vi "collectResults.vi"(6 "Images to Collect":i32, 8 "error in (no error)":errorcluster, 9 "Enum":T1(ring), 10 "ImageData":T2, 11 "ImageAnalyser in":refnum<class "ImageAnalyser.lvclass">) -> (0 "error out":errorcluster, 2 "finished?":bool, 3 "ImageAnalyser out":refnum<class "ImageAnalyser.lvclass">)   [LabVIEW 2011, in "Tools.lvlib" / "Imaging.lvlib" / "ImageAnalyser.lvclass"]
uses:
  ImageAnalyser.lvclass
  ImageAnalyser.lvclass/ImageAnalyser.ctl
  AbsorptionAnalyser/AbsorptionAnalyser.lvclass
  FluorescenceAnalyser/FluorescenceAnalyser.lvclass
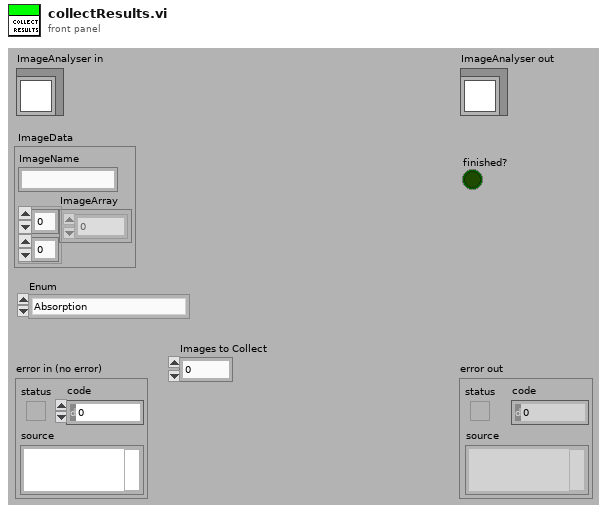
[diagram p1: front panel]
types:
  T1 = enum16{"Absorption", "Fluorescence", "Light Sheet", "Dark Ground"}
  T2 = cluster{"ImageName":string, "ImageArray":sgl[][]}
  T3 = cluster{"Name":string, "Results":dbl[], "AnalysisType":string}
  T4 = cluster{"Name":string, "Results":dbl[], "AnalysisType":string}[]
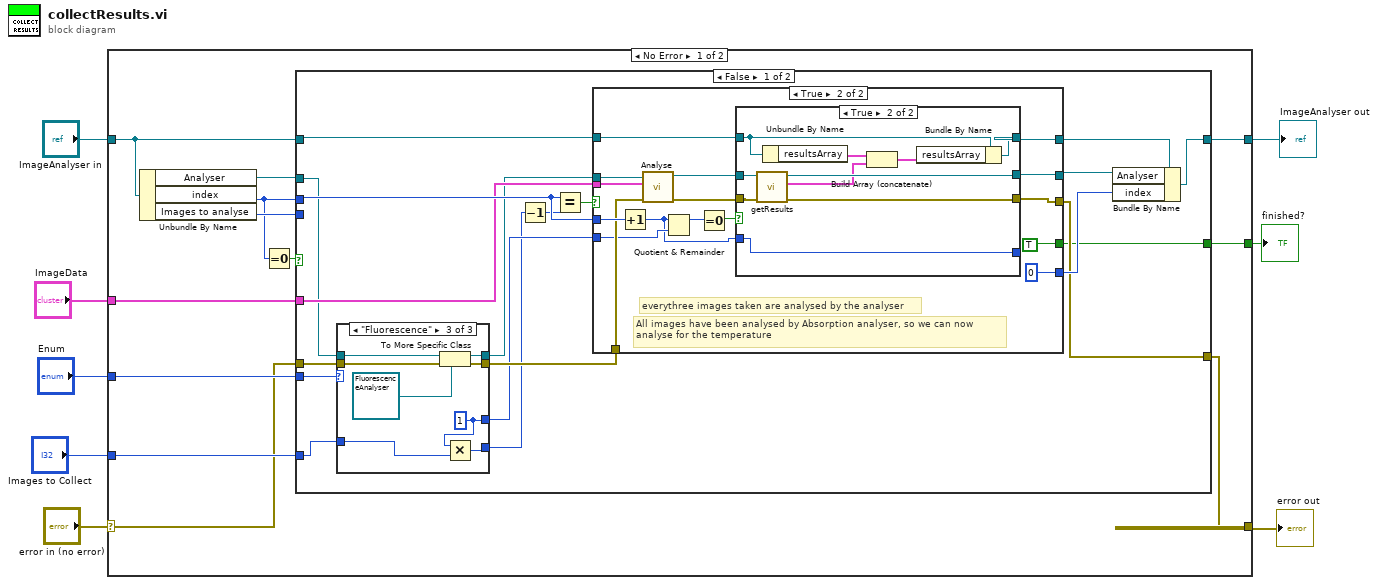
[diagram p0: block diagram]
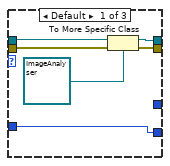
[diagram p2: hidden frame]
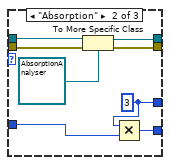
[diagram p3: hidden frame]
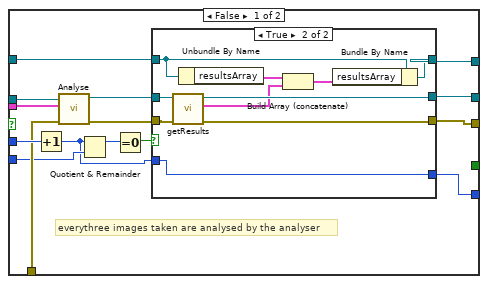
[diagram p4: hidden frame]
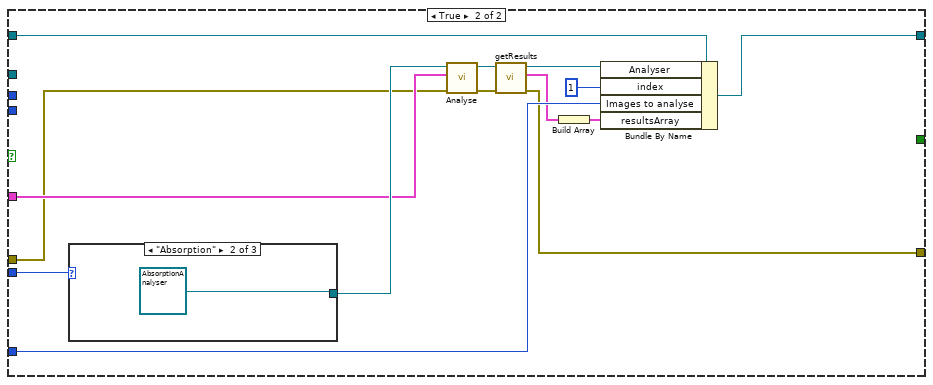
[diagram p7: hidden frame]
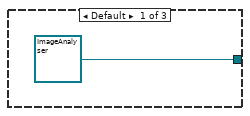
[diagram p8: hidden frame]
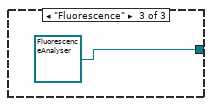
[diagram p9: hidden frame]
diagram:
  n1 = case shown="No Error" "error in (no error)" {
    selector: "error in (no error)" -> [w11 w139]
    tunnel: [w10 w139] -> w7
    tunnel: [w18 w138] -> w5
    tunnel: "ImageAnalyser in" -> [w17 w138]
    tunnel: "Images to Collect" -> [w12 _]
    tunnel: "Enum" -> [w13 _]
    tunnel: "ImageData" -> [w14 _]
    tunnel: [w9 _] -> w1
    frame No Error {
      n2 = Unbundle By Name(w17) -> ("Analyser"=w20:refnum<class>, "index"=w16:i32, "Images to analyse"=w19:i32)
      n3 = Equal To 0?(x=w16) -> (x = 0?=w15:bool)
      n4 = case shown="False" w15 {
        tunnel: w20 -> [w30 _]
        tunnel: w19 -> [_ _]
        tunnel: [w35 w127] -> w18
        tunnel: w17 -> [w34 w134]
        tunnel: w16 -> [w33 _]
        tunnel: w14 -> [w32 w131]
        tunnel: w13 -> [w31 w133]
        tunnel: w12 -> [w23 w129]
        tunnel: w11 -> [w28 w122]
        tunnel: [w26 w121] -> w10
        tunnel: [w24 _] -> w9
        frame False {
          n5 = case shown="\"Fluorescence\"" w31 {
            tunnel: w30 -> [w45 w53 w61]
            tunnel: [w43 w51 w59] -> w29
            tunnel: w28 -> [w41 w50 w58]
            tunnel: [w42 w49 w57] -> w27
            tunnel: [_ w48 w55] -> w25
            tunnel: w23 -> [w40 w47 w54]
            tunnel: [w40 w46 w56] -> w22
            frame Default {
              n6 = To More Specific Class(target class=refnum<class "ImageAnalyser.lvclass"> refnum ("Tools.lvlib:Imaging.lvlib:ImageAnalyser.lvclass"), reference=w45, error in=w41) -> (specific class reference=w43:refnum<class "ImageAnalyser.lvclass">, error out=w42:errorcluster)
            }
            frame "Absorption" {
              w48 = 3
              n7 = To More Specific Class(target class=refnum<class "AbsorptionAnalyser.lvclass"> refnum ("Tools.lvlib:Imaging.lvlib:AbsorptionAnalyser.lvclass"), reference=w53, error in=w50) -> (specific class reference=w51:refnum<class "AbsorptionAnalyser.lvclass">, error out=w49:errorcluster)
              n8 = Multiply(x=w48, y=w47) -> (x*y=w46:i32)
            }
            frame "Fluorescence" {
              w55 = 1
              n9 = To More Specific Class(target class=refnum<class "FluorescenceAnalyser.lvclass"> refnum ("Tools.lvlib:Imaging.lvlib:FluorescenceAnalyser.lvclass"), reference=w61, error in=w58) -> (specific class reference=w59:refnum<class "FluorescenceAnalyser.lvclass">, error out=w57:errorcluster)
              n10 = Multiply(x=w55, y=w54) -> (x*y=w56:i32)
            }
          }
          n11 = Decrement(x=w22) -> (x-1=w21:i32)
          n12 = Equal?(x=w33, y=w21) -> (x = y?=w38:bool)
          n13 = case shown="True" w38 {
            tunnel: w32 -> [w76 w106]
            tunnel: w27 -> [w65 w95]
            tunnel: w29 -> [w75 w105]
            tunnel: [w70 w100] -> w39
            tunnel: [w66 w96] -> w26
            tunnel: [w68 w98] -> w37
            tunnel: w34 -> [w69 w99]
            tunnel: w33 -> [w74 w104]
            tunnel: [w62 0] -> w36
            tunnel: w25 -> [w64 w94]
            tunnel: [_ TRUE] -> w24
            frame False {
              # "everythree images taken are analysed by the analyser"
              n14 = Increment(x=w74) -> (x+1=w63:i32)
              n15 = call-dynamic "Analyse.vi"("error in (no error)"=w65, "ImageData"=w76, "ImageAnalyser in"=w75) -> ("error out"=w67:errorcluster, "ImageAnalyser out"=w72:refnum<class "ImageAnalyser.lvclass">)  [unwired: 7 in]
              n16 = Quotient & Remainder(x=w63, y=w64) -> (x-y*floor(x/y)=w73:i32)  [unwired: 1 out]
              n17 = Equal To 0?(x=w73) -> (x = 0?=w71:bool)
              n18 = case shown="True" w71 {
                tunnel: w72 -> [w80 w86]
                tunnel: [w80 w84] -> w70
                tunnel: w69 -> [w79 w90]
                tunnel: [w79 w89] -> w68
                tunnel: w67 -> [w78 w85]
                tunnel: [w78 w83] -> w66
                tunnel: w63 -> [w77 w81]
                tunnel: [w77 w81] -> w62
                frame False {
                }
                frame True {
                  n19 = call "getResults.vi"("error in (no error)"=w85, "ImageAnalyser in"=w86) -> ("error out"=w83:errorcluster, "results"=w82:T3, "ImageAnalyser out"=w84:refnum<class "ImageAnalyser.lvclass">)  [unwired: 7 in]
                  n20 = Unbundle By Name(w90) -> ("resultsArray"=w88:T4)
                  n21 = Build Array (concatenate)(w88, w82) -> (w87:T4)
                  n22 = Bundle By Name(cluster=w90, "resultsArray"=w87) -> (w89:refnum<class "ImageAnalyser.lvclass">)
                }
              }
            }
            frame True {
              # "All images have been analysed by Absorption analyser, so we can now\nanalyse for the temperature"
              # "everythree images taken are analysed by the analyser"
              n23 = Increment(x=w104) -> (x+1=w93:i32)
              n24 = call-dynamic "Analyse.vi"("error in (no error)"=w95, "ImageData"=w106, "ImageAnalyser in"=w105) -> ("error out"=w97:errorcluster, "ImageAnalyser out"=w102:refnum<class "ImageAnalyser.lvclass">)  [unwired: 7 in]
              n25 = Quotient & Remainder(x=w93, y=w94) -> (x-y*floor(x/y)=w103:i32)  [unwired: 1 out]
              n26 = Equal To 0?(x=w103) -> (x = 0?=w101:bool)
              n27 = case shown="True" w101 {
                tunnel: w102 -> [w110 w116]
                tunnel: [w110 w114] -> w100
                tunnel: w99 -> [w109 w120]
                tunnel: [w109 w119] -> w98
                tunnel: w97 -> [w108 w115]
                tunnel: [w108 w113] -> w96
                tunnel: w93 -> [w107 w111]
                tunnel: [w107 w111] -> _
                frame False {
                }
                frame True {
                  n28 = call "getResults.vi"("error in (no error)"=w115, "ImageAnalyser in"=w116) -> ("error out"=w113:errorcluster, "results"=w112:T3, "ImageAnalyser out"=w114:refnum<class "ImageAnalyser.lvclass">)  [unwired: 7 in]
                  n29 = Unbundle By Name(w120) -> ("resultsArray"=w118:T4)
                  n30 = Build Array (concatenate)(w118, w112) -> (w117:T4)
                  n31 = Bundle By Name(cluster=w120, "resultsArray"=w117) -> (w119:refnum<class "ImageAnalyser.lvclass">)
                }
              }
            }
          }
          n32 = Bundle By Name(cluster=w37, "Analyser"=w39, "index"=w36) -> (w35:refnum<class "ImageAnalyser.lvclass">)
        }
        frame True {
          n33 = case shown="\"Absorption\"" w133 {
            tunnel: [refnum<class "ImageAnalyser.lvclass"> refnum ("Tools.lvlib:Imaging.lvlib:ImageAnalyser.lvclass") refnum<class "AbsorptionAnalyser.lvclass"> refnum ("Tools.lvlib:Imaging.lvlib:AbsorptionAnalyser.lvclass") refnum<class "FluorescenceAnalyser.lvclass"> refnum ("Tools.lvlib:Imaging.lvlib:FluorescenceAnalyser.lvclass")] -> w132
            frame Default {
            }
            frame "Absorption" {
            }
            frame "Fluorescence" {
            }
          }
          n34 = call-dynamic "Analyse.vi"("error in (no error)"=w122, "ImageData"=w131, "ImageAnalyser in"=w132) -> ("error out"=w125:errorcluster, "ImageAnalyser out"=w126:refnum<class "ImageAnalyser.lvclass">)  [unwired: 7 in]
          n35 = call "getResults.vi"("error in (no error)"=w125, "ImageAnalyser in"=w126) -> ("error out"=w121:errorcluster, "results"=w123:T3, "ImageAnalyser out"=w124:refnum<class "ImageAnalyser.lvclass">)  [unwired: 7 in]
          n36 = Build Array(w123) -> (w128:T4)
          n37 = Bundle By Name(cluster=w134, "Analyser"=w124, "index"=1, "Images to analyse"=w129, "resultsArray"=w128) -> (w127:refnum<class "ImageAnalyser.lvclass">)
        }
      }
    }
    frame Error {
    }
  }
  "error out" <- w7
  "ImageAnalyser out" <- w5
  "finished?" <- w1
